vi "4-1.vi"(8 "error in (no error)":errorcluster, 9 "Min Temp.":dbl, 10 "Max Temp.":dbl, 11 "Current Temp.":dbl) -> (0 "error out":errorcluster, 1 "Warning?":bool, 2 "?":string)   [LabVIEW 2014]
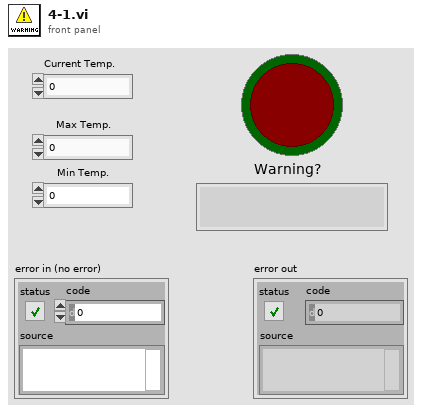
[diagram p1: front panel]
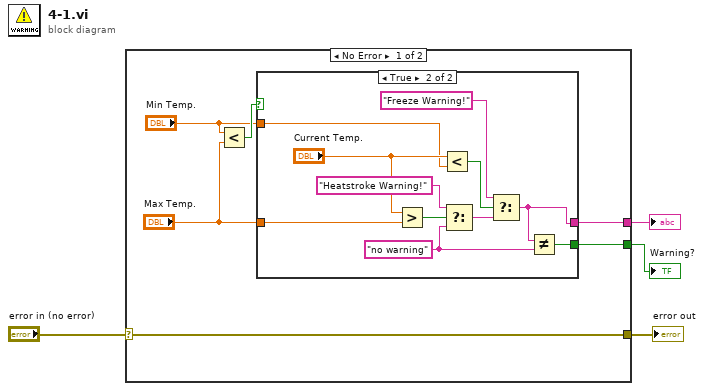
[diagram p0: block diagram]
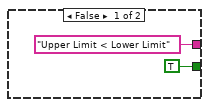
[diagram p2: hidden frame]
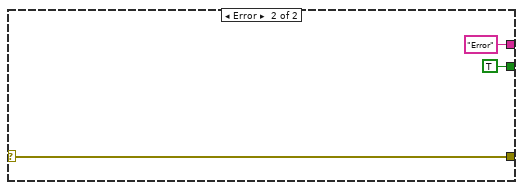
[diagram p3: hidden frame]
diagram:
  n1 = case shown="No Error" "error in (no error)" {
    selector: "error in (no error)" -> [w8 w26]
    tunnel: [w8 w26] -> w3
    tunnel: [w6 "Error"] -> w2
    tunnel: [w5 TRUE] -> w1
    frame No Error {
      n2 = Less?(x="Min Temp.", y="Max Temp.") -> (x < y?=w10:bool)
      n3 = case shown="True" w10 {
        tunnel: [TRUE w22] -> w5
        tunnel: ["Upper Limit < Lower Limit" w19] -> w6
        tunnel: "Max Temp." -> [_ w17]
        tunnel: "Min Temp." -> [_ w14]
        frame False {
        }
        frame True {
          w23 = "no warning"
          n4 = Greater?(x="Current Temp.", y=w17) -> (0:w16:bool)
          n5 = Less?(x="Current Temp.", y=w14) -> (x < y?=w13:bool)
          n6 = Select(t="Heatstroke Warning!", s=w16, f=w23) -> (s? t:f=w18:string)
          n7 = Select(t="Freeze Warning!", s=w13, f=w18) -> (s? t:f=w19:string)
          n8 = Not Equal?(x=w19, y=w23) -> (x != y?=w22:bool)
        }
      }
    }
    frame Error {
    }
  }
  "error out" <- w3
  "?" <- w2
  "Warning?" <- w1
